vi "Write IsOpen.vi"(8 "error in (no error)":errorcluster, 10 "IsOpen":bool, 11 "PIDController in":refnum<class "PIDController.lvclass">) -> (0 "error out":errorcluster, 3 "PIDController out":refnum<class "PIDController.lvclass">)   [LabVIEW 2023, in "PIDController.lvclass"]
uses:
  PIDController.lvclass
  PIDController.lvclass/PIDController.ctl
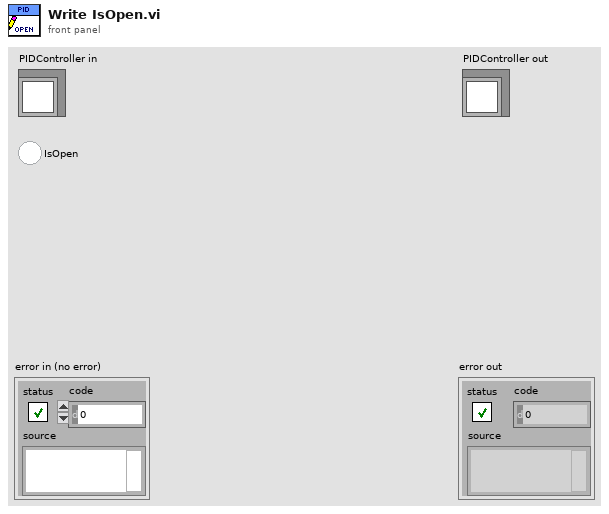
[diagram p1: front panel]
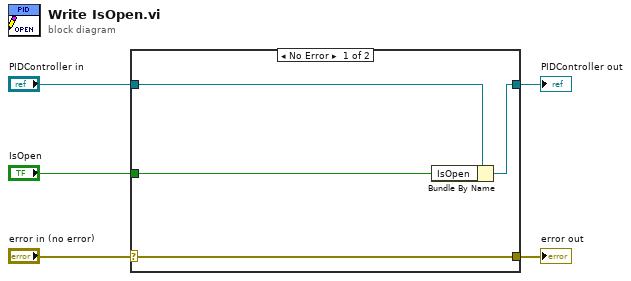
[diagram p0: block diagram]
diagram:
  n1 = case shown="No Error" "error in (no error)" {
    selector: "error in (no error)" -> [w9 w10]
    tunnel: [w9 w10] -> w4
    tunnel: [w7 w11] -> w2
    tunnel: "PIDController in" -> [w8 w11]
    tunnel: "IsOpen" -> [w6 _]
    frame No Error {
      n2 = Bundle By Name(cluster=w8, "IsOpen"=w6) -> (w7:refnum<class "PIDController.lvclass">)
    }
    frame Error {
    }
  }
  "error out" <- w4
  "PIDController out" <- w2
